vi "Get lines and values from string.vi"(3 "Array size":i32, 4 "Input string":string) -> (14 "Numerical values":dbl[](array[numeric]) format="%.2f", 15 "Strings":string[](array[string]), 16 "Item name":string[](array[string]))   [LabVIEW 2020]
doc: "This VI returns numerical values and single lines from input string without any axis assignment. If number of lines/values (Array size) is known, algorithm is faster, otherwise Array size = 0 should be used. Sub-VI for VST?.vi and STE?.vi."
panel:
  # "This vi returns numerical values and/or single lines from input string without any axis assignment. If number \nof lines/values (Array size) is known, algorithm is faster, otherwise Array size = 0 should be used."
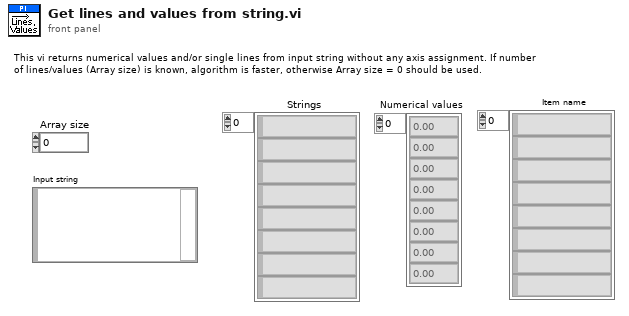
[diagram p1: front panel]
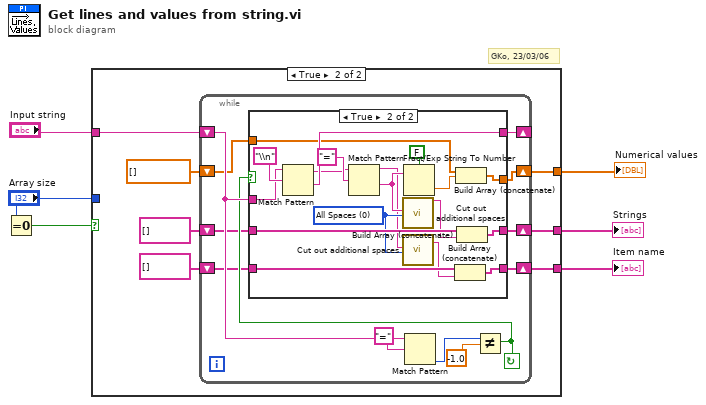
[diagram p0: block diagram]
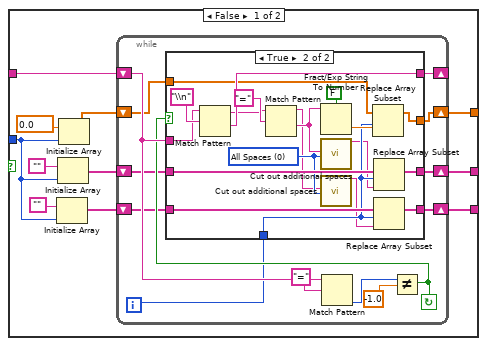
[diagram p2: hidden frame]
diagram:
  # "GKo, 23/03/06"
  n1 = Equal To 0?(x="Array size") -> (x = 0?=w2:bool)
  n2 = case shown="True" w2 {
    tunnel: [w17 w60] -> w6
    tunnel: "Input string" -> [w16 w59]
    tunnel: "Array size" -> [w7 _]
    tunnel: [w11 w58] -> w3
    tunnel: [w10 w55] -> w1
    frame False {
      n3 = Initialize Array("", w7) -> (w9:string[])
      n4 = Initialize Array("", w7) -> (w13:string[])
      n5 = Initialize Array(0.0 ("Element Data"), w7) -> (w14:dbl[])
      n6 = while {
        shift-left: w13 -> [w20]
        shift-right: [w21] -> w11
        shift-left: w14 -> [w24]
        shift-right: [w23] -> w17
        shift-left: w16 -> [w27]
        shift-right: [w26] -> _
        shift-right: [w19] -> w10
        shift-left: w9 -> [w18]
        i -> [w22]
        stop <- w25 continue-if-true
        n7 = Match Pattern(string=w27, regular expression="=") -> (offset past match=w28:i32)  [unwired: 4 out]
        n8 = Not Equal?(x=w28, y=-1.0) -> (x != y?=w25:bool)
        n9 = case shown="True" w25 {
          tunnel: w27 -> [w34 w52]
          tunnel: [w34 w51] -> w26
          tunnel: [w33 w49] -> w23
          tunnel: w24 -> [w33 w50]
          tunnel: w22 -> [_ w40]
          tunnel: [w32 w44] -> w21
          tunnel: w20 -> [w32 w43]
          tunnel: [w31 w42] -> w19
          tunnel: w18 -> [w31 w41]
          frame False {
          }
          frame True {
            w39 = u16 0 items=["All Spaces", "Only if 1st char.", "Only if last char.", "Only if near \"=\""] ("Mode")
            n10 = Match Pattern(string=w52, regular expression="\\n") -> (before substring=w46:string, after substring=w51:string)  [unwired: 3 out]
            n11 = Match Pattern(string=w46, regular expression="=") -> (before substring=w36:string, after substring=w38:string)  [unwired: 3 out]
            n12 = Fract/Exp String To Number(use system decimal point (T)=FALSE, string=w38) -> (number=w45:dbl)  [unwired: 3 out]
            n13 = call "Cut out additional spaces.vi"("String"=w38, "Mode"=w39) -> ("String out"=w37:string)  [unwired: 17 out]
            n14 = call "Cut out additional spaces.vi"("String"=w36, "Mode"=w39) -> ("String out"=w35:string)  [unwired: 17 out]
            n15 = Replace Array Subset(array=w50, new element=w45, index=w40) -> (w49:dbl[])
            n16 = Replace Array Subset(array=w43, new element=w37, index=w40) -> (w44:string[])
            n17 = Replace Array Subset(array=w41, new element=w35, index=w40) -> (w42:string[])
          }
        }
      }
    }
    frame True {
      n18 = while {
        shift-left: string[] [] -> [w63]
        shift-right: [w64] -> w58
        shift-left: dbl[] [] -> [w66]
        shift-right: [w65] -> w60
        shift-left: w59 -> [w69]
        shift-right: [w68] -> _
        shift-right: [w62] -> w55
        shift-left: string[] [] -> [w61]
        stop <- w67 continue-if-true
        n19 = Match Pattern(string=w69, regular expression="=") -> (offset past match=w70:i32)  [unwired: 4 out]
        n20 = Not Equal?(x=w70, y=-1.0) -> (x != y?=w67:bool)
        n21 = case shown="True" w67 {
          tunnel: w69 -> [w76 w93]
          tunnel: [w76 w92] -> w68
          tunnel: [w75 w90] -> w65
          tunnel: w66 -> [w75 w91]
          tunnel: [w74 w86] -> w64
          tunnel: w63 -> [w74 w85]
          tunnel: [w73 w81] -> w62
          tunnel: w61 -> [w73 w80]
          frame False {
          }
          frame True {
            w79 = u16 0 items=["All Spaces", "Only if 1st char.", "Only if last char.", "Only if near \"=\""] ("Mode")
            n22 = Match Pattern(string=w93, regular expression="\\n") -> (before substring=w87:string, after substring=w92:string)  [unwired: 3 out]
            n23 = Match Pattern(string=w87, regular expression="=") -> (before substring=w78:string, after substring=w83:string)  [unwired: 3 out]
            n24 = call "Cut out additional spaces.vi"("String"=w83, "Mode"=w79) -> ("String out"=w82:string)  [unwired: 17 out]
            n25 = call "Cut out additional spaces.vi"("String"=w78, "Mode"=w79) -> ("String out"=w77:string)  [unwired: 17 out]
            n26 = Fract/Exp String To Number(use system decimal point (T)=FALSE, string=w83) -> (number=w84:dbl)  [unwired: 3 out]
            n27 = Build Array (concatenate)(w80, w77) -> (w81:string[])
            n28 = Build Array (concatenate)(w91, w84) -> (w90:dbl[])
            n29 = Build Array (concatenate)(w85, w82) -> (w86:string[])
          }
        }
      }
    }
  }
  "Numerical values" <- w6
  "Strings" <- w3
  "Item name" <- w1
